vi "archivedGUI_HallProbe1.0.0.vi"() -> ()   [LabVIEW 2020]
panel:
  out "indecator ref array":refnum<vi>[](array[refnum])
  in  "time to wait (TCP) 2":i32=10
  in  "plot":bool=TRUE
  out "ratio(h)":bool
  out "fixsize":bool
  in  "shotnumber":i32
  out "error (h)":bool
  out "Device Name (h)":string="unknown"
  in  "Main Tap":T1(tab)
  in  "Field":dbl
  out "local Port":u16=65455
  out "port or service name":u16=65454
  out "Remote Host":string="192.168.10.157"
  in  "timeout ms (slow resp)":i32=500
  in  "reset":bool
  out "image con closed":bool
  out "image \nconnection":bool
  out "image con closed 2":bool
  out "All Devices (h)":string[](array[string])=["StagingHallProbe"]
  in  "time to wait (TCP)":i32=10
  out "error out":errorcluster
  out "connections (hidden)":variant[](array[variant])=[variant(refnum<k16> refnum), variant(refnum<k16> refnum)]
  in  "time to wait (main loop)":i32=10
  out "Data String":string
  in  "Local Saving Path":path
  out "error message":string
  out "Data Connection out":bool
  # "(mT)"
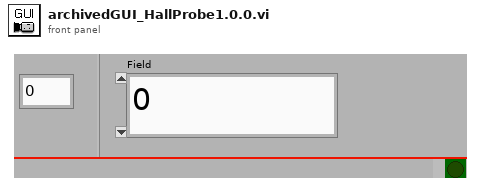
[diagram p1: front panel]
types:
  T1 = enum32{"All Channels", "Network", "Internal", "Advanced"}
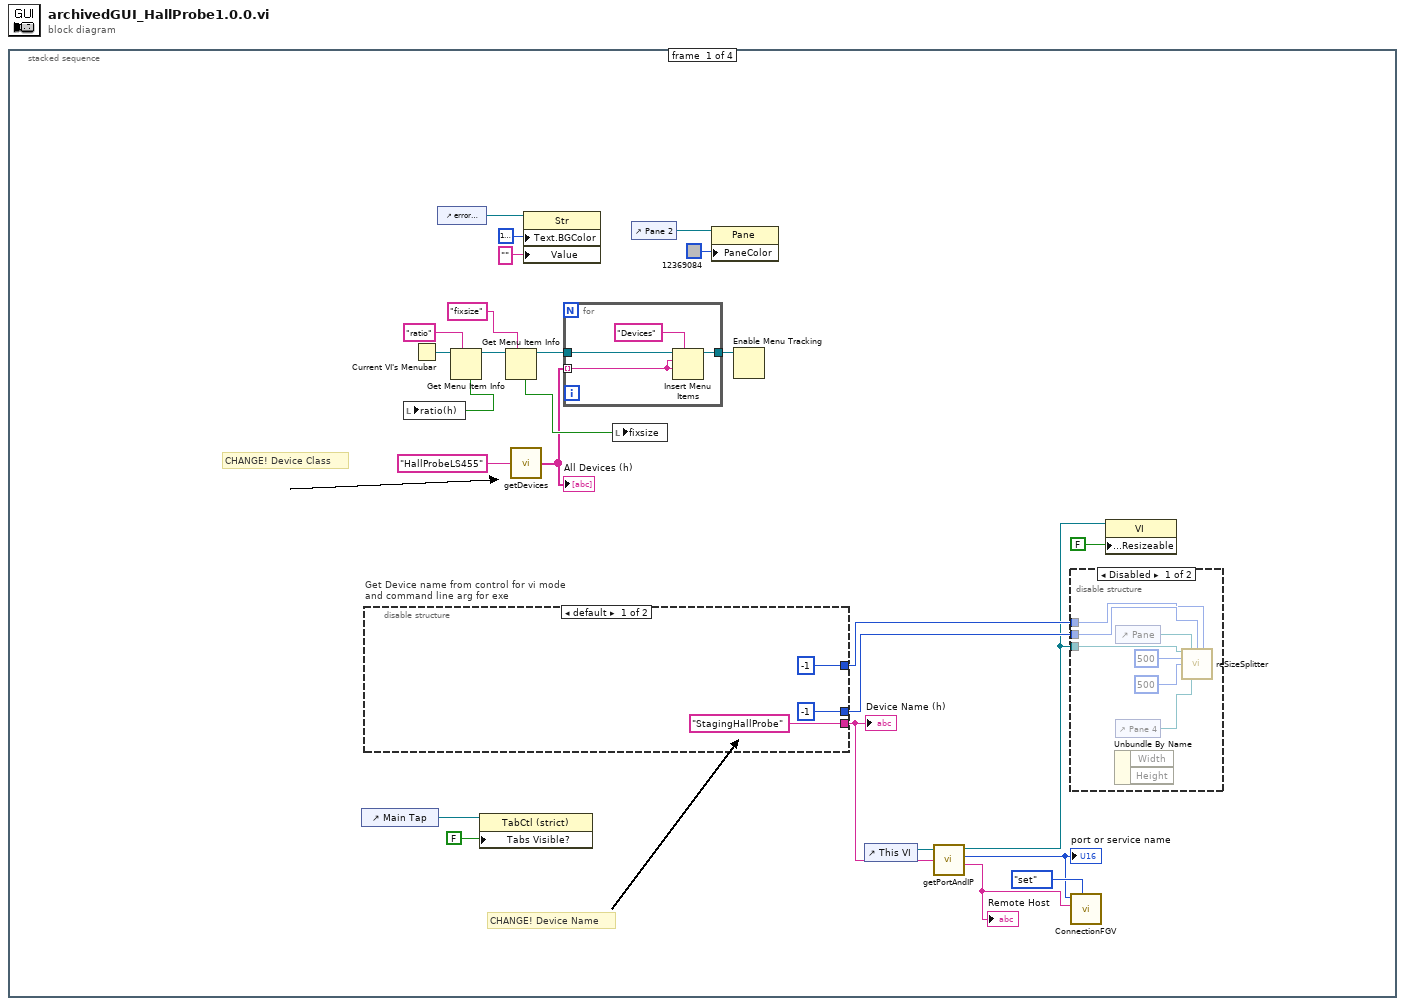
[diagram p0: block diagram]
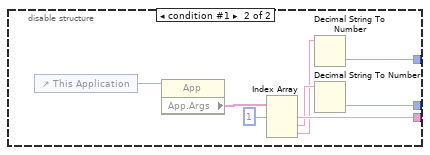
[diagram p3: hidden frame]
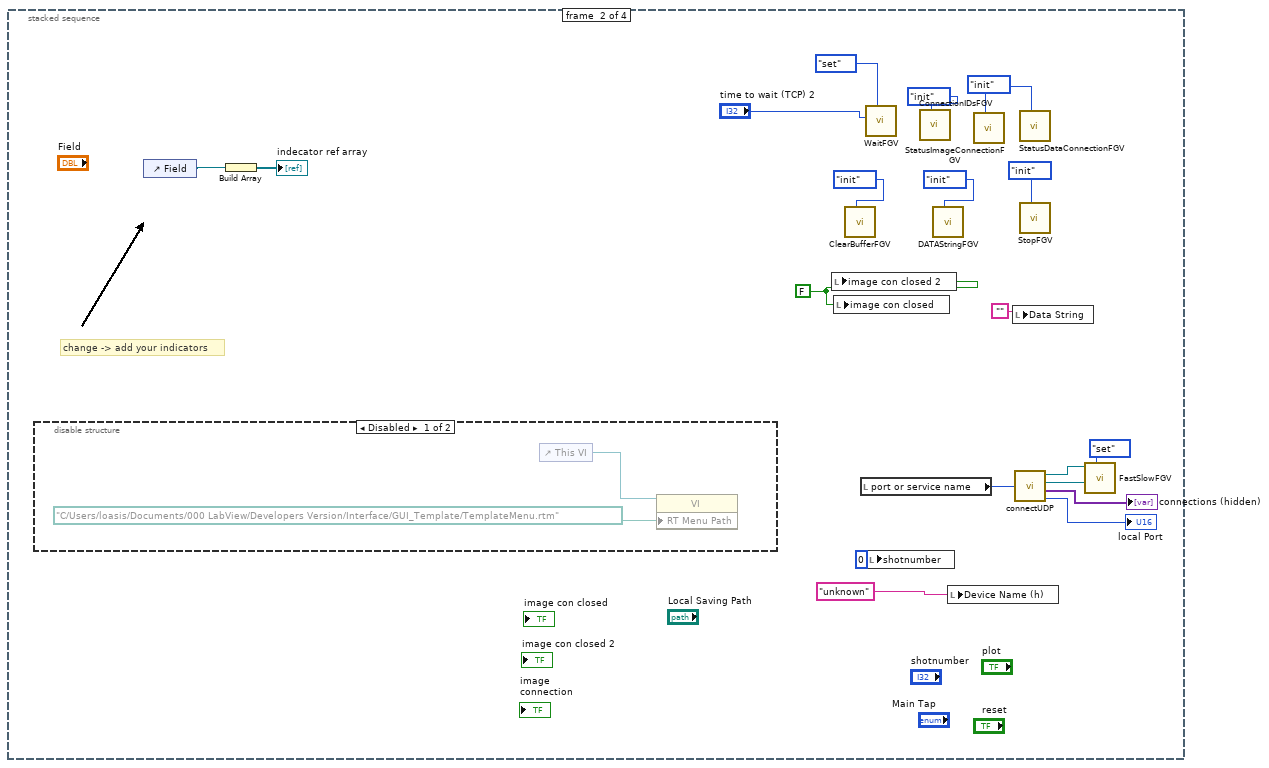
[diagram p4: hidden frame]
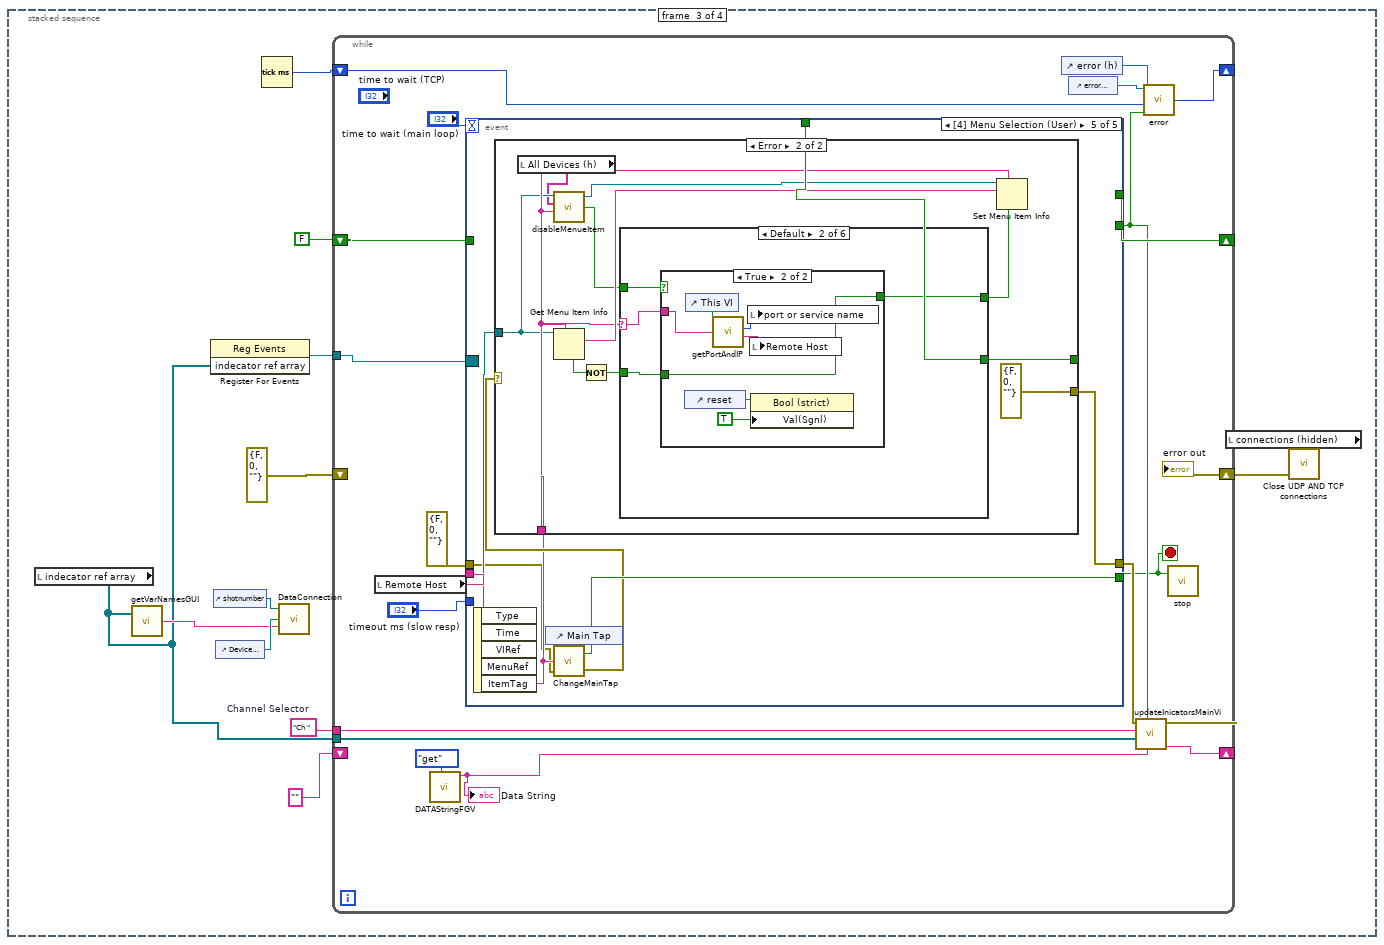
[diagram p6: hidden frame]
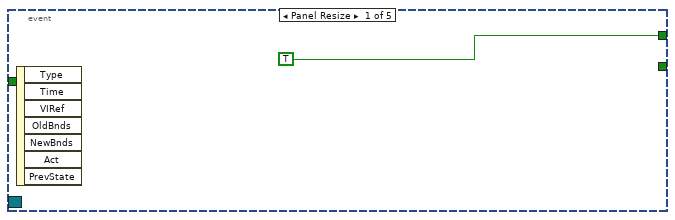
[diagram p7: hidden frame]
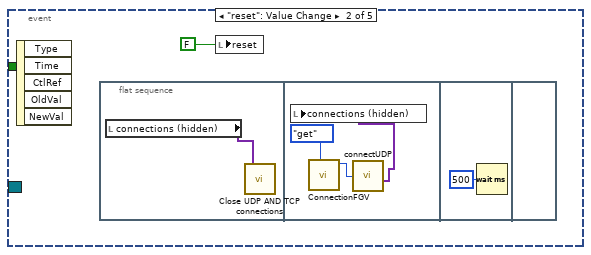
[diagram p8: hidden frame]
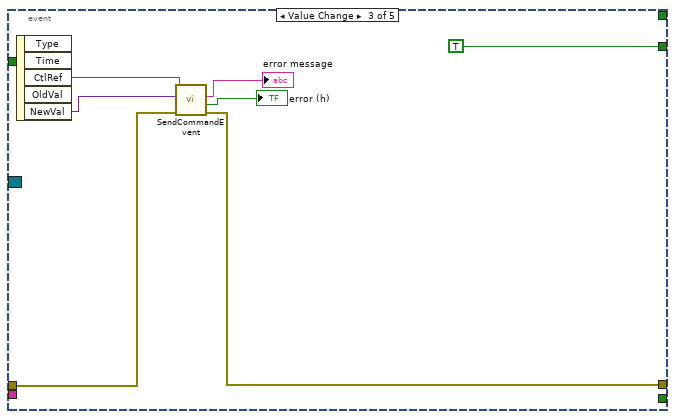
[diagram p9: hidden frame]
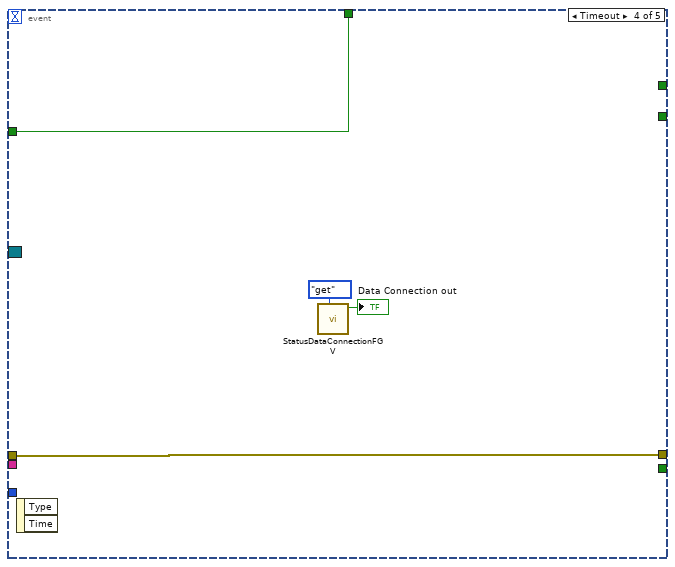
[diagram p10: hidden frame]
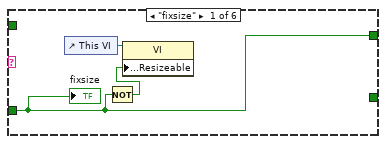
[diagram p12: hidden frame]
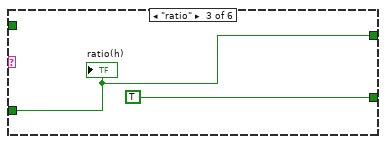
[diagram p14: hidden frame]
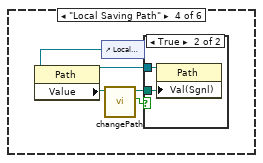
[diagram p15: hidden frame]
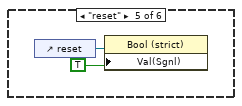
[diagram p17: hidden frame]
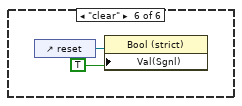
[diagram p18: hidden frame]
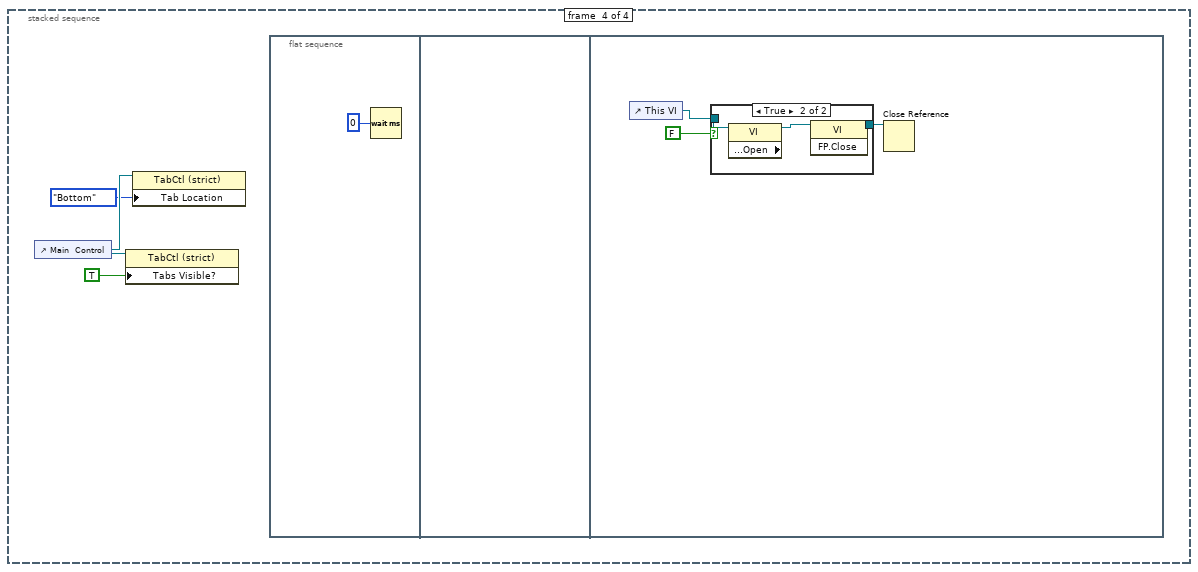
[diagram p19: hidden frame]
diagram:
  n1 = stacked-sequence {
    frame #0 {
      # "CHANGE! Device Name"
      # "CHANGE! Device Class"
      n2 = control-ref of="Main Tap"() -> (w26:refnum<vi>)
      n3 = disable-structure "Get Device name from control for vi mode\nand command line arg for exe" shown="default" {
        disable-tunnel: ["StagingHallProbe" ("Device Name for vi mode") w45] -> w22
        disable-tunnel: [i16 -1 ("left") w42] -> w24
        disable-tunnel: [i16 -1 ("left") w41] -> w23
        frame condition #0 (active) {
        }
        frame condition #1 {
          n4 = control-ref of="This Application"() -> (w48:refnum<vi>)
          n5 = property class="App"(reference=w48) -> ("App.Args"=w47:string[])  [unwired: 1 in, 2 out]
          n6 = Index Array(array=w47, index #1=1 ("index")) -> (element #1=w45:string, element #2=w44:string, element #3=w43:string)  [unwired: 2 in]
          n7 = Decimal String To Number(string=w43) -> (number=w41:i32)  [unwired: 2 in, 1 out]
          n8 = Decimal String To Number(string=w44) -> (number=w42:i32)  [unwired: 2 in, 1 out]
        }
      }
      "Device Name (h)" <- w22
      n9 = Current VI's Menubar() -> (w14:refnum<k9>)
      n10 = control-ref of="error message"() -> (w8:refnum<vi>)
      n11 = Get Menu Item Info(7:"ratio" ("item tag"), 11:w14) -> (3:w12:refnum<k9>, 4:w13:bool)  [unwired: 1 in, 5 out]
      n12 = local write "ratio(h)"(w13) -> ()
      n13 = property class="TabCtl (strict)"(reference=w26, "Tabs Visible?"=FALSE) -> ()  [unwired: 1 in, 2 out]
      n14 = Get Menu Item Info(7:"fixsize" ("item tag"), 11:w12) -> (3:w4:refnum<k9>, 4:w10:bool)  [unwired: 1 in, 5 out]
      n15 = call "getDevices.vi"("Device Class"="HallProbeLS455") -> ("All Devices"=w2:string[])
      "All Devices (h)" <- w2
      n16 = property class="Str"(reference=w8, "Text.BGColor"=u32 16777238, "Value"="") -> ()  [unwired: 1 in, 2 out]
      n17 = for {
        tunnel: w4 -> [w30]
        tunnel: [w29] -> w3
        tunnel: w2 -> [w27] mode=indexing
        n18 = Insert Menu Items(5:"Devices" ("menu tag"), 7:w27, 8:w27, 9:w30) -> (3:w29:refnum<k9>)  [unwired: 2 in, 2 out]
      }
      n19 = local write "fixsize"(w10) -> ()
      n20 = control-ref of="Pane 2"() -> (w6:refnum<vi>)
      n21 = property class="Pane"(reference=w6, "PaneColor"=u32 12369084) -> ()  [unwired: 1 in, 2 out]
      n22 = Enable Menu Tracking(4:w3) -> ()  [unwired: 2 in, 2 out]
      n23 = control-ref of="This VI"() -> (w21:refnum<vi>)
      n24 = call "getPortAndIP.vi"("Device Name"=w22, "This Vi"=w21) -> ("Remote Host"=w17:string, "port or service name"=w16:u16, "reference out"=w19:refnum<vi>)  [unwired: 2 in, 2 out]
      "port or service name" <- w16
      "Remote Host" <- w17
      n25 = disable-structure shown="Disabled" {
        disable-tunnel: w24 -> [w36 _]
        disable-tunnel: w23 -> [w35 _]
        disable-tunnel: w19 -> [w33 _]
        frame Disabled {
          n26 = Unbundle By Name() -> ()  [unwired: 1 in, 2 out]
          n27 = control-ref of="Pane"() -> (w37:refnum<vi>)
          n28 = control-ref of="Pane 4"() -> (w34:refnum<vi>)
          n29 = call "reSizeSplitter.vi"("this vi"=w33, "pane"=w37, "left"=w36, "top"=w35, "Width"=u32 500, "Height"=u32 500, "pane2"=w34) -> ()  [unwired: 8 in, 1 out]
        }
        frame Enabled {
        }
      }
      n30 = call "ConnectionFGV.vi"("command"=enum16{"get", "set", "init"}."set", "Remote Host in"=w17, "port or service name in"=w16) -> ()  [unwired: 7 in, 2 out]
      n31 = property class="VI"(reference=w19, "Front Panel.Resizeable"=FALSE ("Front Panel Window:Resizable")) -> ()  [unwired: 1 in, 2 out]
    }
    frame #1 {
      w59 = enum16{"get", "set", "init"}."init" ("Command")
      w65 = FALSE ("new Device Data")
      # "change -> add your indicators"
      n32 = disable-structure shown="Disabled" {
        frame Disabled {
          n33 = control-ref of="This VI"() -> (w69:refnum<vi>)
          n34 = property class="VI"(reference=w69, "RT Menu Path"=path "C:/Users/loasis/Documents/000 LabView/Developers Version/Interface/GUI_Template/TemplateMenu.rtm" ("Run-Time Menu Path")) -> ()  [unwired: 1 in, 2 out]
        }
        frame Enabled {
        }
      }
      n35 = control-ref of="Field"() -> (w49:refnum<vi>)
      n36 = Build Array(w49) -> (→"indecator ref array":refnum<vi>[])
      n37 = local write "image con closed 2"(w65) -> ()
      n38 = local write "image con closed"(w65) -> ()
      n39 = call "ClearBufferFGV.vi"("Command"=enum16{"set", "get", "init"}."init") -> ()  [unwired: 10 in, 1 out]
      n40 = local read "port or service name"() -> (w55:u16)
      n41 = call "WaitFGV.vi"("Command"=enum16{"get", "set", "init"}."set", "milliseconds to wait"="time to wait (TCP) 2") -> ()  [unwired: 9 in, 1 out]
      n42 = local write "shotnumber"(0 ("shotnumber")) -> ()
      n43 = call "ConnectionIDsFGV.vi"("Command"=enum16{"add", "get", "init"}."init") -> ()  [unwired: 10 in, 1 out]
      n44 = call "DATAStringFGV.vi"("Command"=enum16{"get", "set", "init"}."init") -> ()  [unwired: 9 in, 2 out]
      n45 = local write "Device Name (h)"("unknown" ("Device Name")) -> ()
      n46 = call "StatusImageConnectionFGV.vi"("Command"=w59) -> ()  [unwired: 10 in, 1 out]
      n47 = local write "Data String"("") -> ()
      n48 = call "connectUDP.vi"("port or service name NOT USED"=w55) -> ("fast ID (h)"=w54:refnum<k16>, "slow ID (h)"=w53:refnum<k16>, "connections (hidden)"=→"connections (hidden)":variant[], "local Port"=→"local Port":u16)
      n49 = call "StatusDataConnectionFGV.vi"("Command"=w59) -> ()  [unwired: 10 in, 1 out]
      n50 = call "StopFGV.vi"("Command"=enum16{"set", "get", "init"}."init") -> ()  [unwired: 9 in, 2 out]
      n51 = call "FastSlowFGV.vi"("Command"=enum16{"get", "set", "init"}."set", "slow ID"=w53, "fast ID"=w54) -> ()  [unwired: 7 in, 2 out]
    }
    frame #2 {
      w72 = "Ch "  # Channel Selector
      n52 = local read "indecator ref array"() -> (w70:refnum<vi>[])
      n53 = call "getVarNamesGUI.vi"("Array"=w70) -> ("String"=w71:string)  [unwired: 1 in]
      n54 = register-events(w70) -> (reference out=w73:refnum<event-registration>)  [unwired: 2 in, 1 out]
      n55 = control-ref of="shotnumber"() -> (w75:refnum<vi>)
      n56 = control-ref of="Device Name (h)"() -> (w74:refnum<vi>)
      n57 = Tick Count (ms)() -> (millisecond timer value=w77:u32)
      n58 = call "DataConnection.vi"("Subscriber list"=w71, "Device Name (h)"=w74, "shotnumber"=w75) -> ()
      n59 = while {
        shift-right: [w97] -> w80
        shift-left: errorcluster {"status"=FALSE, "code"=0, "source"=""} ("error out") -> [_]
        tunnel: w70 -> [w91]
        shift-right: [w95] -> _
        shift-left: FALSE -> [w96]
        shift-right: [w94] -> _
        shift-left: w77 -> [w93]
        shift-right: [w84] -> _
        shift-left: "" ("Data String") -> [_]
        tunnel: w73 -> [w87]
        tunnel: w72 -> [w86]
        stop <- w88 stop-if-true
        n60 = local read "Remote Host"() -> (w99:string)
        n61 = call "DATAStringFGV.vi"("Command"=enum16{"get", "set", "init"}."get") -> ("Data String out"=w89:string)  [unwired: 9 in, 1 out]
        "Data String" <- w89
        n62 = event shown="[4] Menu Selection (User)" {
          selector: w87 -> [_ _ _ _ _]
          dyn-events: _ -> [_ _ _ _ _]
          timeout: "time to wait (main loop)" -> [_ _ _ _ _]
          tunnel: [_ _ w113 w119 w121] -> w98
          tunnel: w99 -> [_ _ _ _ _]
          tunnel: "timeout ms (slow resp)" -> [_ _ _ _ _]
          tunnel: errorcluster {"status"=FALSE, "code"=0, "source"=""} ("error out") -> [_ _ w110 w119 w122]
          tunnel: [_ _ TRUE _ _] -> w92
          tunnel: [_ _ _ _ w127] -> w88
          tunnel: [_ _ _ w118 w124] -> _
          tunnel: w96 -> [_ _ _ w118 _]
          tunnel: [TRUE _ _ _ _] -> w95
          event Panel Resize {
            n63 = event-data() -> ()  [unwired: 1 in, 7 out]
          }
          event "reset": Value Change {
            n64 = event-data() -> ()  [unwired: 1 in, 5 out]
            n65 = flat-sequence {
              frame #0 {
                n66 = local read "connections (hidden)"() -> (w104:variant[])
                n67 = call "Close UDP AND TCP connections.vi"("appended array"=w104) -> ()  [unwired: 7 in]
              }
              frame #1 {
                n68 = call "ConnectionFGV.vi"("command"=enum16{"get", "set", "init"}."get") -> ("port or service name out"=w106:u16)  [unwired: 9 in, 1 out]
                n69 = call "connectUDP.vi"("port or service name NOT USED"=w106) -> ("connections (hidden)"=w105:variant[])  [unwired: 3 out]
                n70 = local write "connections (hidden)"(w105) -> ()
              }
              frame #2 {
                n71 = Wait (ms)(milliseconds to wait=u32 500) -> ()  [unwired: 1 out]
              }
              frame #3 {
              }
            }
            n72 = local write "reset"(FALSE ("reset")) -> ()
          }
          event Value Change {
            n73 = event-data() -> ("CtlRef"=w115:refnum<vi>, "NewVal"=w114:variant)  [unwired: 1 in, 3 out]
            n74 = call "SendCommandEvent.vi"("error out 2"=w110, "NewVal"=w114, "CtlRef"=w115) -> ("error out"=w113:errorcluster, "error (h)"=→"error (h)":bool, "error message"=→"error message":string)  [unwired: 5 in, 1 out]
          }
          event Timeout {
            n75 = event-data() -> ()  [unwired: 1 in, 2 out]
            n76 = call "StatusDataConnectionFGV.vi"("Command"=enum16{"get", "set", "init"}."get") -> ("Data Connection out"=→"Data Connection out":bool)  [unwired: 10 in]
          }
          event Menu Selection (User) {
            n77 = event-data() -> ("MenuRef"=w123:refnum<k9>, "ItemTag"=w125:string)  [unwired: 1 in, 3 out]
            n78 = control-ref of="Main Tap"() -> (w120:refnum<vi>)
            n79 = call "ChangeMainTap.vi"("error in"=w122, "ItemTag"=w125, "reference"=w120) -> ("error out"=w126:errorcluster, "Boolean"=w127:bool)
            n80 = case shown="Error" w126 {
              selector: w126 -> [w128 _]
              tunnel: w123 -> [_ w134]
              tunnel: [_ w136] -> w124
              tunnel: w125 -> [_ w135]
              tunnel: [w128 errorcluster {"status"=FALSE, "code"=0, "source"=""} ("error IO")] -> w121
              frame No Error {
              }
              frame Error {
                n81 = local read "All Devices (h)"() -> (w129:string[])
                n82 = call "disableMenueItem.vi"("ItemTag"=w135, "All Devices (h)"=w129, "MenuRef"=w134) -> ("this is a Device(tag)"=w133:bool, "menu reference out"=w132:refnum<k9>)  [unwired: 1 in, 1 out]
                n83 = Get Menu Item Info(7:w135, 11:w134) -> (2:w138:string, 4:w139:bool)  [unwired: 1 in, 5 out]
                n84 = Not(x=w139) -> (.not. x?=w137:bool)
                n85 = case shown="Default" w135 {
                  selector: w135 -> [_ w145 _ _ _ _]
                  tunnel: w137 -> [w140 w143 w154 _ _ _]
                  tunnel: [_ _ TRUE _ _ _] -> w136
                  tunnel: w133 -> [_ w146 _ _ _ _]
                  tunnel: [w140 w144 w154 _ _ _] -> w131
                  frame "fixsize" {
                    n86 = control-ref of="This VI"() -> (w142:refnum<vi>)
                    n87 = Not(x=w140) -> (.not. x?=w141:bool)
                    n88 = property class="VI"(reference=w142, "Front Panel.Resizeable"=w141) -> ()  [unwired: 1 in, 2 out]
                    "fixsize" <- w140
                  }
                  frame Default {
                    n89 = case shown="True" w146 {
                      tunnel: w145 -> [_ w153]
                      tunnel: [_ w147] -> w144
                      tunnel: w143 -> [_ w147]
                      frame False {
                      }
                      frame True {
                        n90 = control-ref of="reset"() -> (w149:refnum<vi>)
                        n91 = control-ref of="This VI"() -> (w152:refnum<vi>)
                        n92 = call "getPortAndIP.vi"("Device Name"=w153, "This Vi"=w152) -> ("Remote Host"=w151:string, "port or service name"=w150:u16)  [unwired: 2 in, 3 out]
                        n93 = local write "port or service name"(w150) -> ()
                        n94 = local write "Remote Host"(w151) -> ()
                        n95 = property class="Bool (strict)"(reference=w149, "Val(Sgnl)"=TRUE ("Value (Signaling)")) -> ()  [unwired: 1 in, 2 out]
                      }
                    }
                  }
                  frame "ratio" {
                    "ratio(h)" <- w154
                  }
                  frame "Local Saving Path" {
                    n96 = control-ref of="Local Saving Path"() -> (w156:refnum<vi>)
                    n97 = property class="Path"(reference=w156) -> (reference out=w159:refnum<vi>, "Value"=w160:path)  [unwired: 1 in, 1 out]
                    n98 = call "changePath.vi"("Local Saving in (h)"=w160) -> ("change (h)"=w158:bool, "Local Saving out (h)"=w157:path)  [unwired: 9 in]
                    n99 = case shown="True" w158 {
                      tunnel: w159 -> [_ w162]
                      tunnel: w157 -> [_ w161]
                      frame False {
                      }
                      frame True {
                        n100 = property class="Path"(reference=w162, "Val(Sgnl)"=w161) -> ()  [unwired: 1 in, 2 out]
                      }
                    }
                  }
                  frame "reset" {
                    n101 = control-ref of="reset"() -> (w164:refnum<vi>)
                    n102 = property class="Bool (strict)"(reference=w164, "Val(Sgnl)"=TRUE ("Value (Signaling)")) -> ()  [unwired: 1 in, 2 out]
                  }
                  frame "clear" {
                    n103 = control-ref of="reset"() -> (w166:refnum<vi>)
                    n104 = property class="Bool (strict)"(reference=w166, "Val(Sgnl)"=TRUE ("Value (Signaling)")) -> ()  [unwired: 1 in, 2 out]
                  }
                }
                n105 = Set Menu Item Info(6:w131, 7:w135, 10:w138, 11:w132) -> ()  [unwired: 3 in, 2 out]
              }
            }
          }
        }
        n106 = control-ref of="error (h)"() -> (w82:refnum<vi>)
        n107 = control-ref of="error message"() -> (w83:refnum<vi>)
        n108 = call "updateInicatorsMainVi.vi"("Data String out"=w89, "Boolean"=w92, "Array"=w91, "Channel Selector"=w86, "error in"=w98) -> ("Data String out 2"=w84:string, "error out"=w97:errorcluster)  [unwired: 4 in, 1 out]
        "error out" <- w97
        n109 = call "error.vi"("Boolean"=w92, "millisecond timer value"=w93, "reference"=w82, "error message"=w83) -> ("millisecond timer value 2"=w94:u32)
        n110 = call "stop.vi"("Boolean"=w88) -> ()
      }
      n111 = local read "connections (hidden)"() -> (w79:variant[])
      n112 = call "Close UDP AND TCP connections.vi"("error in"=w80, "appended array"=w79) -> ()  [unwired: 6 in]
    }
    frame #3 {
      n113 = control-ref of="Main  Control"() -> (w168:refnum<vi>)
      n114 = property class="TabCtl (strict)"(reference=w168, "Tabs Visible?"=TRUE) -> ()  [unwired: 1 in, 2 out]
      n115 = property class="TabCtl (strict)"(reference=w168, "Tab Location"=enum32{"Top", "Bottom", "Left", "Right"}."Bottom") -> ()  [unwired: 1 in, 2 out]
      n116 = flat-sequence {
        frame #0 {
          n117 = Wait (ms)(milliseconds to wait=u32 0) -> ()  [unwired: 1 out]
        }
        frame #1 {
        }
        frame #2 {
          n118 = control-ref of="This VI"() -> (w173:refnum<vi>)
          n119 = case shown="True" FALSE {
            tunnel: w173 -> [w174 w177]
            tunnel: [w174 w175] -> w172
            frame False {
            }
            frame True {
              n120 = property class="VI" props=["Front Panel.Open"](reference=w177) -> (reference out=w176:refnum<vi>)  [unwired: 1 in, 2 out]
              n121 = invoke class="VI" method="FP.Close"(reference=w176) -> (reference out=w175:refnum<vi>)  [unwired: 2 in, 2 out]
            }
          }
          n122 = Close Reference(reference=w172) -> ()  [unwired: 1 in, 1 out]
        }
      }
    }
  }
